vi "hw3_4.vi"() -> ()   [LabVIEW 2014]
panel:
  out "combinations":i32[][](array[numeric])
  in  "n steps":i32
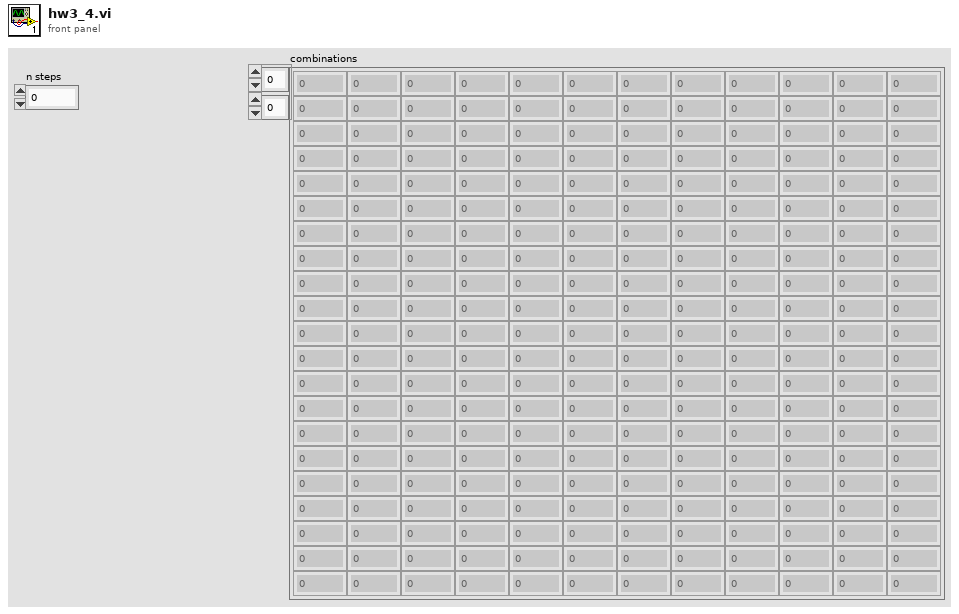
[diagram p1: front panel]
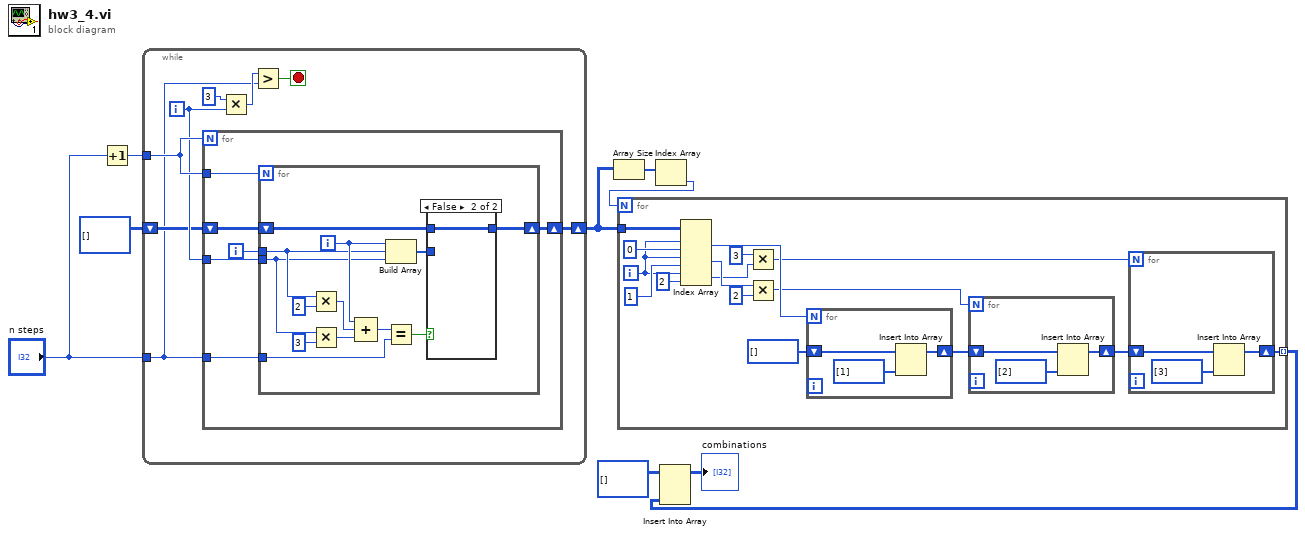
[diagram p0: block diagram]
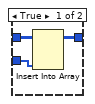
[diagram p2: hidden frame]
diagram:
  n1 = Increment(x="n steps") -> (x+1=w9:i32)
  n2 = while {
    tunnel: w9 -> [w16]
    tunnel: "n steps" -> [w10]
    shift-right: [w14] -> w2
    shift-left: i32[][] [] -> [w13]
    i -> [w15]
    stop <- w17 stop-if-true
    n3 = for {
      N: w16 -> [_]
      tunnel: w16 -> [w23]
      tunnel: w15 -> [w21]
      tunnel: w10 -> [w20]
      shift-right: [w19] -> w14
      shift-left: w13 -> [w18]
      i -> [w22]
      n4 = for {
        N: w23 -> [_]
        tunnel: w22 -> [w27]
        tunnel: w21 -> [w26]
        tunnel: w20 -> [w30]
        shift-right: [w24] -> w19
        shift-left: w18 -> [w29]
        i -> [w28]
        n5 = Multiply(x=w27, y=2) -> (x*y=w33:i32)
        n6 = Multiply(x=w26, y=3) -> (x*y=w35:i32)
        n7 = Compound Arithmetic op=ADD(w28, w33, w35) -> (w36:i32)
        n8 = Build Array(w28, w27, w26) -> (w25:i32[])
        n9 = Equal?(x=w36, y=w30) -> (x = y?=w31:bool)
        n10 = case shown="False" w31 {
          tunnel: w29 -> [w39 w40]
          tunnel: [w38 w40] -> w24
          tunnel: w25 -> [w37 _]
          frame True {
            n11 = Insert Into Array(array=w39, new element=w37) -> (w38:i32[][])  [unwired: 2 in]
          }
          frame False {
          }
        }
      }
    }
    n12 = Multiply(x=3, y=w15) -> (x*y=w11:i32)
    n13 = Greater?(x=w11, y=w10) -> (0:w17:bool)
  }
  n14 = Array Size(array=w2) -> (size(s)=w4:i32[])
  n15 = Index Array(array=w4) -> (element=w1:i32)  [unwired: 1 in]
  n16 = for {
    N: w1 -> [_]
    tunnel: [w56] -> w3 mode=indexing
    tunnel: w2 -> [w52]
    i -> [w46]
    n17 = Index Array(array=w52, index (row) #1=w46, index (col) #1=0 ("disabled index (col)"), index (row) #2=w46, index (col) #2=1 ("disabled index (col)"), index (row) #3=w46, index (col) #3=2 ("disabled index (col)")) -> (element #1=w48:i32, element #2=w47:i32, element #3=w41:i32)
    n18 = Multiply(x=3 ("y"), y=w41) -> (x*y=w43:i32)
    n19 = Multiply(x=w47, y=2) -> (x*y=w45:i32)
    n20 = for {
      N: w48 -> [_]
      shift-right: [w63] -> w55
      shift-left: i32[] [] -> [w64]
      n21 = Insert Into Array(array=w64, new element=i32[] [1]) -> (w63:i32[])  [unwired: 1 in]
    }
    n22 = for {
      N: w45 -> [_]
      shift-right: [w60] -> w54
      shift-left: w55 -> [w61]
      n23 = Insert Into Array(array=w61, new element=i32[] [2]) -> (w60:i32[])  [unwired: 1 in]
    }
    n24 = for {
      N: w43 -> [_]
      shift-right: [w57] -> w56
      shift-left: w54 -> [w58]
      n25 = Insert Into Array(array=w58, new element=i32[] [3]) -> (w57:i32[])  [unwired: 1 in]
    }
  }
  n26 = Insert Into Array(array=i32[][] [], new element=w3) -> (→"combinations":i32[][])  [unwired: 2 in]
